vi "Set Change Type to Modify on Parent.vi"(10 "parent name":string, 11 "refresh items in":T1[](array[typedef])) -> (3 "refresh items out":T1[](array[typedef]))   [LabVIEW 2020, in "Ballard MIL-STD-1553 System Explorer.lvlib" / "Implementation.lvlib" / "Refresh.lvlib"]
uses:
  Refresh.lvlib
  MCL Row.ctl
  Change Type.ctl
  Symbols.ctl
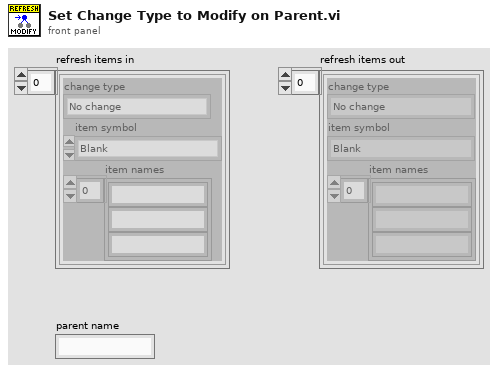
[diagram p1: front panel]
types:
  T1 = typedef "Ballard MIL-STD-1553 System Explorer.lvlib/Implementation.lvlib/Refresh.lvlib/MCL Row.ctl" = cluster{"change type":T2, "item symbol":T3, "item names":string[]}
  T2 = typedef "Ballard MIL-STD-1553 System Explorer.lvlib/Implementation.lvlib/Refresh.lvlib/Change Type.ctl" = enum16{"No change", "Modify", "Add", "Remove"}
  T3 = typedef "Ballard MIL-STD-1553 System Explorer.lvlib/Implementation.lvlib/Refresh.lvlib/Symbols.ctl" = enum16{"Blank", "MIL-STD-1553", "Port", "Remote Terminal", "Subaddress", "Bus Controller", "Acyclic Frame", "Mode Code", "Message", "Parameter", "Item"}
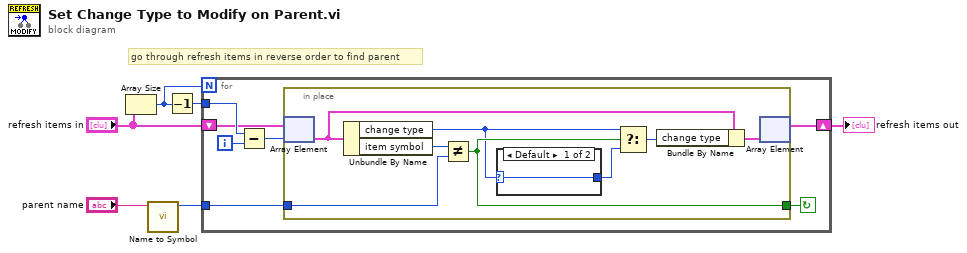
[diagram p0: block diagram]
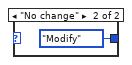
[diagram p2: hidden frame]
diagram:
  # "go through refresh items in reverse order to find parent"
  n1 = Array Size(array="refresh items in") -> (size(s)=w5:i32)
  n2 = call "Name to Symbol.vi"("item name"="parent name") -> ("item symbol"=w1:T3)  [unwired: 10 in]
  n3 = Decrement(x=w5) -> (x-1=w4:i32)
  n4 = for {
    N: w5 -> [_]
    tunnel: w1 -> [w13]
    shift-right: [w7] -> w3
    shift-left: "refresh items in" -> [w9]
    tunnel: w4 -> [w10]
    i -> [w11]
    stop <- w12 continue-if-true
    n5 = Subtract(x=w10, y=w11) -> (x-y=w8:i32)
    n6 = in-place {
      in-place-border: w13 -> [w21]
      in-place-border: [w20] -> w12
      n7 = in-place-array #1(w9, w8) -> (w19:T1)
      n8 = Unbundle By Name(w19) -> ("change type"=w14:T2, "item symbol"=w15:T3)
      n9 = Not Equal?(x=w15, y=w21) -> (x != y?=w20:bool)
      n10 = case shown="Default" w14 {
        selector: w14 -> [w22 _]
        tunnel: [w22 Change_Type."Modify" ("t")] -> w17
        frame Default {
        }
        frame "No change" {
        }
      }
      n11 = Select(t=w14, s=w20, f=w17) -> (s? t:f=w16:T2)
      n12 = Bundle By Name(cluster=w19, "change type"=w16) -> (w18:T1)
      n13 = in-place-array #1(w18) -> (w7:T1[])  [unwired: 1 out]
    }
  }
  "refresh items out" <- w3
